vi "启停.vi"(8 "error in (no error)":errorcluster, 11 "启停":u16(ring) items=["停止", "启动"]) -> (0 "error out":errorcluster)   [LabVIEW 2016, in "DR803M4.lvlib"]
uses:
  DR803M4.lvlib
  <vilib>/Plasmionique/MB Master/MB_Master_Serial/MB_Master_Serial.lvclass
  C:/Program Files (x86)/National Instruments/LabVIEW 2016/vi.lib/Plasmionique/MB Master/MB_Master/MB_Master.lvclass
  Global variable/input variable.vi
  <vilib>/Plasmionique/MB Master/MB Master.lvlib
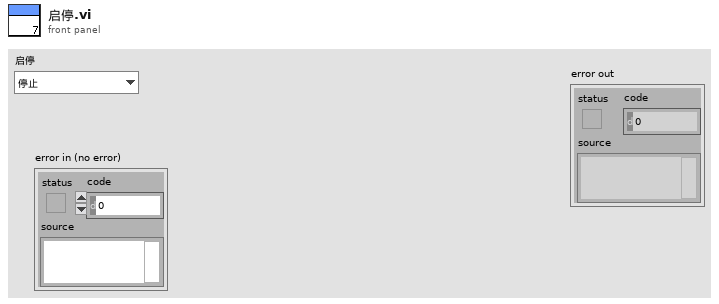
[diagram p1: front panel]
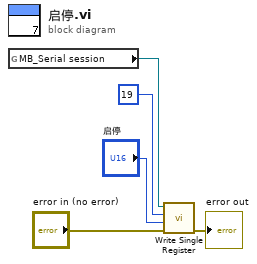
[diagram p0: block diagram]
diagram:
  n1 = global read "input variable.vi" "MB_Serial session"() -> (w5:refnum<class "MB_Master_Serial.lvclass">)
  n2 = call <vilib>:"Write Single Register.vi"("error in (no error)"="error in (no error)", "value"="启停", "address"=u16 19, "MB session in"=w5) -> ("error out"=→"error out":errorcluster)  [unwired: 6 in, 1 out]
